vi "ActionVIOnCompile.vi"(8 "error in (no error)":errorcluster, 11 "Device Item Ref in":T1 format="%.0x") -> (0 "error out":errorcluster)   [LabVIEW 2020, in "AIM MIL-STD-1553 System Explorer.lvlib"]
uses:
  AIM MIL-STD-1553 System Explorer.lvlib
  <vilib>/NI VeriStand/Custom Device API/Custom Device API.lvlib
  Includes/AIM MIL-STD-1553 Engine.lvlibp/Engine/Implementation/Execution Unit Factory/Execution Unit Factory.lvclass
  Includes/AIM MIL-STD-1553 Engine.lvlibp/Engine/Implementation/Shared Resources Factory/Shared Resources Factory.lvclass
  Includes/AIM MIL-STD-1553 Engine.lvlibp/Engine/Interfaces/Execution Unit Factory/Execution Unit Factory.lvclass
  Includes/AIM MIL-STD-1553 Engine.lvlibp/Engine/Interfaces/Shared Resources Factory/Shared Resources Factory.lvclass
  Includes/AIM MIL-STD-1553 Engine.lvlibp/1abvi3w/vi.lib/NI VeriStand/Custom Device API/Data Reference.ctl
  Includes/AIM MIL-STD-1553 Engine.lvlibp/1abvi3w/vi.lib/NI VeriStand/Custom Device API/Block Data Reference.ctl
  Includes/AIM MIL-STD-1553 Engine.lvlibp/Engine/Custom Device/Inline Execution Unit Compiled Information.ctl
  Includes/AIM MIL-STD-1553 Engine.lvlibp/Engine/Custom Device/Asynchronous Execution Unit Compiled Information.ctl
  Includes/AIM MIL-STD-1553 Engine.lvlibp/Engine/Custom Device/Compiled.Settings.ctl
  <vilib>/NI VeriStand/Custom Device API/Set Item Property (Variant).vi
  <vilib>/Utility/xml.llb/Write to XML File(string).vi
  <vilib>/NI VeriStand/Custom Device API/Custom Device Item Ref.ctl
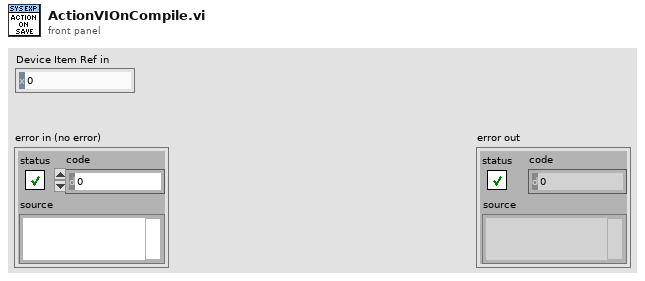
[diagram p1: front panel]
types:
  T1 = typedef "Custom Device API.lvlib/Custom Device Item Ref.ctl" = u64
  T2 = typedef "AIM MIL-STD-1553 System Explorer.lvlibp/Custom Device API.lvlib/Custom Device Item Ref.ctl" = u64
  T3 = typedef "AIM MIL-STD-1553 Engine.lvlibp/Custom Device.lvlib/Compiled.Settings.ctl" = cluster{"Name":string, "Inline Execution Unit Compiled Information":T4[], "Asynchronous Execution Unit Compiled Information":cluster{"Grouped Asynchronous Execution Unit Compiled Information":T7[]}[], "Flattened Shared Resources":string}
  T4 = typedef "AIM MIL-STD-1553 Engine.lvlibp/Custom Device.lvlib/Inline Execution Unit Compiled Information.ctl" = cluster{"Flattened Execution Unit":string, "Incoming Buffer":dbl[], "Outgoing Buffer":dbl[], "Incoming Data References":T5[], "Outgoing Data References":T6[]}
  T5 = typedef "AIM MIL-STD-1553 Engine.lvlibp/Custom Device API.lvlib/Data Reference.ctl" = i32
  T6 = typedef "AIM MIL-STD-1553 Engine.lvlibp/Custom Device API.lvlib/Block Data Reference.ctl" = cluster{"Data Reference":T5, "Offset":u64, "Length":u64}
  T7 = typedef "AIM MIL-STD-1553 Engine.lvlibp/Custom Device.lvlib/Asynchronous Execution Unit Compiled Information.ctl" = cluster{"Flattened Execution Unit":string, "Incoming Channel Group Name":string, "Outgoing Channel Group Name":string, "ReadWrite Channel Group Name":string}
  T8 = typedef "Custom Device API.lvlib/Custom Device Item Info.ctl" = cluster{"Name":string, "Is Channel":bool, "GUID":string, "Is Waveform":bool}
  T9 = typedef "AIM MIL-STD-1553 Engine.lvlibp/Interfaces.lvlib/Execution Unit Information.ctl" = cluster{"Execution Unit":refnum<class "Execution Unit.lvclass">, "Incoming Channels":T10[], "Outgoing Channels":T10[], "ReadWrite Channels":T10[]}
  T10 = typedef "AIM MIL-STD-1553 Engine.lvlibp/Custom Device API.lvlib/Custom Device Item Ref.ctl" = u64
  T11 = cluster{"Grouped Asynchronous Execution Units":T9[]}[]
  T12 = typedef "AIM MIL-STD-1553 Shared.lvlib/Inline Execution Unit Compiled Information.ctl" = cluster{"Flattened Execution Unit":string, "Incoming Buffer":dbl[], "Outgoing Buffer":dbl[], "Incoming Data References":T13[], "Outgoing Data References":T14[]}
  T13 = typedef "Custom Device API.lvlib/Data Reference.ctl" = i32
  T14 = typedef "Custom Device API.lvlib/Block Data Reference.ctl" = cluster{"Data Reference":T13, "Offset":u64, "Length":u64}
  T15 = typedef "AIM MIL-STD-1553 Shared.lvlib/Asynchronous Execution Unit Compiled Information.ctl" = cluster{"Flattened Execution Unit":string, "Incoming Channel Group Name":string, "Outgoing Channel Group Name":string, "ReadWrite Channel Group Name":string}
  T16 = cluster{"Compiled Grouped Asynchronous Execution Units":T15[]}[]
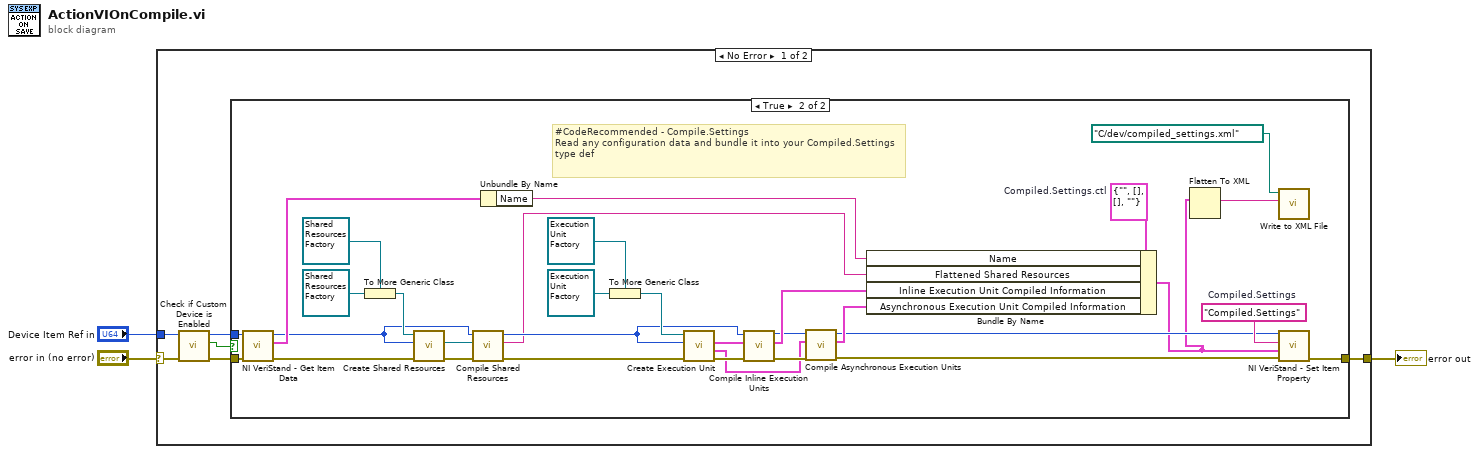
[diagram p0: block diagram]
diagram:
  n1 = case shown="No Error" "error in (no error)" {
    selector: "error in (no error)" -> [w8 w43]
    tunnel: [w9 w43] -> w2
    tunnel: "Device Item Ref in" -> [w6 _]
    frame No Error {
      n2 = call "Check if Custom Device is Enabled.vi"("error in"=w8, "custom device ref"=w6) -> ("error out"=w7:errorcluster, "is enabled?"=w4:bool, "custom device ref out"=w5:T2)  [unwired: 7 in]
      n3 = case shown="True" w4 {
        tunnel: [w10 w41] -> w9
        tunnel: w7 -> [w10 w38]
        tunnel: w5 -> [_ w36]
        frame False {
        }
        frame True {
          w39 = T3 {"Name"="", "Inline Execution Unit Compiled Information"=[], "Asynchronous Execution Unit Compiled Information"=[], "Flattened Shared Resources"=""}  # Compiled.Settings.ctl
          w42 = "Compiled.Settings"  # Compiled.Settings
          # "#CodeRecommended - Compile.Settings\nRead any configuration data and bundle it into your Compiled.Settings type def"
          n4 = call <vilib>:"NI VeriStand - Get Item Data.vi"("error in (no error)"=w38, "Item Ref in"=w36) -> ("error out"=w22:errorcluster, "Item Info"=w40:T8, "Item Ref out"=w18:T1)  [unwired: 6 in, 1 out]
          n5 = To More Generic Class(target class=refnum<class "Shared Resources Factory.lvclass"> refnum ("Interfaces.lvlib:Shared Resources Factory.lvclass"), reference=refnum<class "Shared Resources Factory.lvclass"> refnum ("Implementation.lvlib:Shared Resources Factory.lvclass")) -> (generic class reference=w21:refnum<class "Shared Resources Factory.lvclass">)
          n6 = call-dynamic "Create Shared Resources.vi"("error in"=w22, "custom device ref"=w18, "shared resources factory in"=w21) -> ("error out"=w20:errorcluster, "shared resources"=w19:refnum<class "Shared Resources.lvclass">)  [unwired: 6 in, 1 out]
          n7 = call "Compile Shared Resources.vi"("error in"=w20, "shared resources"=w19, "device ref in"=w18) -> ("error out"=w16:errorcluster, "flattened shared resources"=w14:string, "device ref out"=w17:T1)  [unwired: 6 in]
          n8 = Unbundle By Name(w40) -> ("Name"=w15:string)
          n9 = To More Generic Class(target class=refnum<class "Execution Unit Factory.lvclass"> refnum ("Interfaces.lvlib:Execution Unit Factory.lvclass"), reference=refnum<class "Execution Unit Factory.lvclass"> refnum ("Implementation.lvlib:Execution Unit Factory.lvclass")) -> (generic class reference=w35:refnum<class "Execution Unit Factory.lvclass">)
          n10 = call-dynamic "Create Execution Unit.vi"("error in"=w16, "Item Ref"=w17, "Execution Unit Factory in"=w35) -> ("error out"=w37:errorcluster, "Asynchronous Execution Units"=w27:T11, "Inline Execution Units"=w33:T9[])  [unwired: 5 in, 1 out]
          n11 = call "Compile Inline Execution Units.vi"("error in"=w37, "Inline Execution Units"=w33, "Device Ref in"=w17) -> ("error out"=w32:errorcluster, "Compiled Inline Execution Units"=w34:T12[], "Device Ref out"=w31:T1)  [unwired: 6 in]
          n12 = call "Compile Asynchronous Execution Units.vi"("Device Ref in"=w31, "Asynchronous Execution Units"=w27, "error in"=w32) -> ("Device Ref out"=w28:T1, "Compiled Asynchronous Execution Units"=w30:T16, "error out"=w29:errorcluster)  [unwired: 5 in]
          n13 = Bundle By Name(cluster=w39, "Name"=w15, "Flattened Shared Resources"=w14, "Inline Execution Unit Compiled Information"=w34, "Asynchronous Execution Unit Compiled Information"=w30) -> (w11:T3)
          n14 = Flatten To XML(6:w11) -> (2:w12:string)
          n15 = call-poly <vilib>:"Write to XML File.vi"("XML Input"=w12, "XML File Path"=path "C:/dev/compiled_settings.xml") -> ()  [unwired: 7 in, 3 out]
          n16 = call-poly <vilib>:"NI VeriStand - Set Item Property.vi"("error in (no error)"=w29, "Value"=w11, "Property Name"=w42, "Item Ref in"=w28) -> ("error out"=w41:errorcluster)  [unwired: 5 in, 2 out]
        }
      }
    }
    frame Error {
    }
  }
  "error out" <- w2
